vi "ADO Connection Open Schema.vi"(8 "error in (no error)":errorcluster caption="错误输入（无错误）", 9 "Schema":i32(ring)=-1 items=["adSchemaProviderSpecific"=-1, "adSchemaAsserts"=0, "adSchemaCatalogs"=1, "adSchemaCharacterSets"=2, "adSchemaCollations"=3, "adSchemaColumns"=4, "adSchemaCheckConstraints"=5, "adSchemaConstraintColumnUsage"=6, "adSchemaConstraintTableUsage"=7, "adSchemaKeyColumnUsage"=8, "adSchemaReferentialContraints, adSchemaReferentialConstraints"=9, "adSchemaTableConstraints"=10, "adSchemaColumnsDomainUsage"=11, "adSchemaIndexes"=12, "adSchemaColumnPrivileges"=13, "adSchemaTablePrivileges"=14, "adSchemaUsagePrivileges"=15, "adSchemaProcedures"=16, "adSchemaSchemata"=17, "adSchemaSQLLanguages"=18, "adSchemaStatistics"=19, "adSchemaTables"=20, "adSchemaTranslations"=21, "adSchemaProviderTypes"=22, "adSchemaViews"=23, "adSchemaViewColumnUsage"=24, "adSchemaViewTableUsage"=25, "adSchemaProcedureParameters"=26, "adSchemaForeignKeys"=27, "adSchemaPrimaryKeys"=28, "adSchemaProcedureColumns"=29, "adSchemaDBInfoKeywords"=30, "adSchemaDBInfoLiterals"=31, "adSchemaCubes"=32, "adSchemaDimensions"=33, "adSchemaHierarchies"=34, "adSchemaLevels"=35, "adSchemaMeasures"=36, "adSchemaProperties"=37, "adSchemaMembers"=38, "adSchemaTrustees"=39], 11 "Database Connection 输入":refnum<class "Database Connection.lvclass"> caption="DNL_LabVIEW Object in") -> (0 "error out":errorcluster caption="错误输出", 1 "Schema Data":string[](array[string]), 3 "Database Connection 输出":refnum<class "Database Connection.lvclass"> caption="DNL_LabVIEW Object out")   [LabVIEW 2011, in "Database Connection.lvclass"]
uses:
  Database Connection.lvclass
  Database Connection.lvclass/Database Connection.ctl
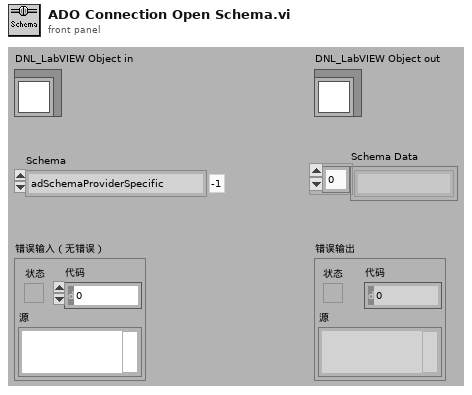
[diagram p1: front panel]
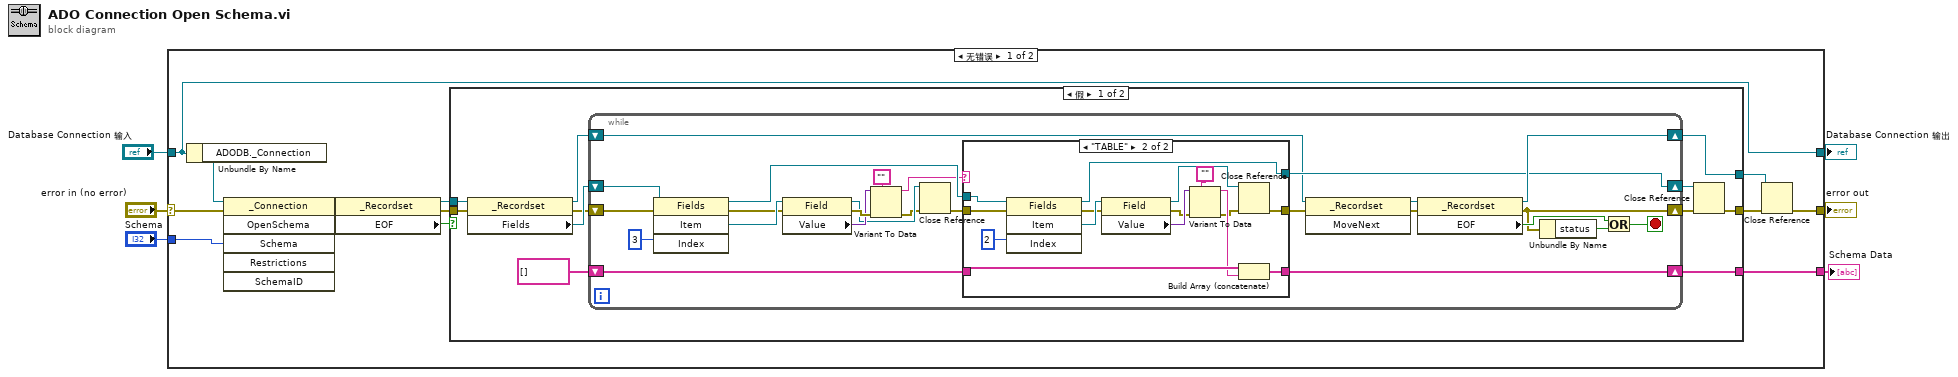
[diagram p0: block diagram]
diagram:
  n1 = case shown="无错误" "error in (no error)" {
    selector: "error in (no error)" -> [w15 w77]
    tunnel: [w8 w77] -> w5
    tunnel: [w19 w76] -> w3
    tunnel: "Database Connection 输入" -> [w19 w76]
    tunnel: "Schema" -> [w17 _]
    tunnel: [w10 _] -> w1
    frame No Error {
      n2 = Unbundle By Name(w19) -> ("ADODB._Connection"=w18:refnum<k7>)
      n3 = invoke class="_Connection" method="OpenSchema"(reference=w18, error in=w15, "Schema"=w17) -> (error out=w14:errorcluster, "OpenSchema"=w16:refnum<k7>)  [unwired: 3 in, 4 out]
      n4 = property class="_Recordset"(reference=w16, error in=w14) -> (reference out=w12:refnum<k7>, error out=w11:errorcluster, "EOF"=w13:bool)
      n5 = case shown="假" w13 {
        tunnel: [w27 _] -> w10
        tunnel: [w24 w74] -> w9
        tunnel: [w22 w75] -> w7
        tunnel: w12 -> [w21 w75]
        tunnel: w11 -> [w20 w74]
        frame False {
          n6 = property class="_Recordset"(reference=w21, error in=w20) -> (reference out=w30:refnum<k7>, error out=w28:errorcluster, "Fields"=w29:refnum<k7>)
          n7 = while {
            shift-right: [w47] -> w23
            shift-left: w29 -> [w55]
            shift-right: [w41] -> w25
            shift-left: w28 -> [w53]
            shift-right: [w50] -> w22
            shift-left: w30 -> [w32]
            shift-right: [w38] -> w27
            shift-left: string[] [] -> [w39]
            stop <- w54 stop-if-true
            n8 = invoke class="Fields" method="Item"(reference=w55, error in=w53, "Index"=3) -> (reference out=w48:refnum<k7>, error out=w31:errorcluster, "Item"=w46:refnum<k7>)  [unwired: 1 in, 1 out]
            n9 = property class="Field"(reference=w46, error in=w31) -> (reference out=w36:refnum<k7>, error out=w44:errorcluster, "Value"=w37:variant)
            n10 = Variant To Data(error in=w44, type="", Variant=w37) -> (data=w33:string, error out=w35:errorcluster)
            n11 = Close Reference(reference=w36, error in (no error)=w35) -> (error out=w34:errorcluster)
            n12 = case shown="\"TABLE\"" w33 {
              tunnel: [w57 w66] -> w38
              tunnel: w48 -> [w58 w72]
              tunnel: [w58 w70] -> w47
              tunnel: [w56 w60] -> w40
              tunnel: w39 -> [w57 w67]
              tunnel: w34 -> [w56 w62]
              frame Default {
              }
              frame "TABLE" {
                n13 = invoke class="Fields" method="Item"(reference=w72, error in=w62, "Index"=2) -> (reference out=w70:refnum<k7>, error out=w69:errorcluster, "Item"=w71:refnum<k7>)  [unwired: 1 in, 1 out]
                n14 = property class="Field"(reference=w71, error in=w69) -> (reference out=w59:refnum<k7>, error out=w63:errorcluster, "Value"=w64:variant)
                n15 = Variant To Data(error in=w63, type="", Variant=w64) -> (data=w65:string, error out=w61:errorcluster)
                n16 = Close Reference(reference=w59, error in (no error)=w61) -> (error out=w60:errorcluster)
                n17 = Build Array (concatenate)(w67, w65) -> (w66:string[])
              }
            }
            n18 = invoke class="_Recordset" method="MoveNext"(reference=w32, error in=w40) -> (reference out=w52:refnum<k7>, error out=w51:errorcluster)  [unwired: 1 in, 1 out]
            n19 = property class="_Recordset"(reference=w52, error in=w51) -> (reference out=w50:refnum<k7>, error out=w41:errorcluster, "EOF"=w42:bool)
            n20 = Unbundle By Name(w41) -> ("status"=w49:bool)
            n21 = Or(x=w42, y=w49) -> (x .or. y?=w54:bool)
          }
          n22 = Close Reference(reference=w23, error in (no error)=w25) -> (error out=w24:errorcluster)
        }
        frame True {
          # "No objects in the database."
        }
      }
      n23 = Close Reference(reference=w7, error in (no error)=w9) -> (error out=w8:errorcluster)
    }
    frame Error {
    }
  }
  "error out" <- w5
  "Database Connection 输出" <- w3
  "Schema Data" <- w1
